vi "AfterLoad.vi"(8 "error in (no error)":errorcluster, 11 "SettingsFile in":refnum<class "SettingsFile.lvclass">) -> (0 "error out":errorcluster, 3 "SettingsFile out":refnum<class "SettingsFile.lvclass">)   [LabVIEW 2018, in "SettingsFile.lvclass"]
uses:
  SettingsFile.lvclass
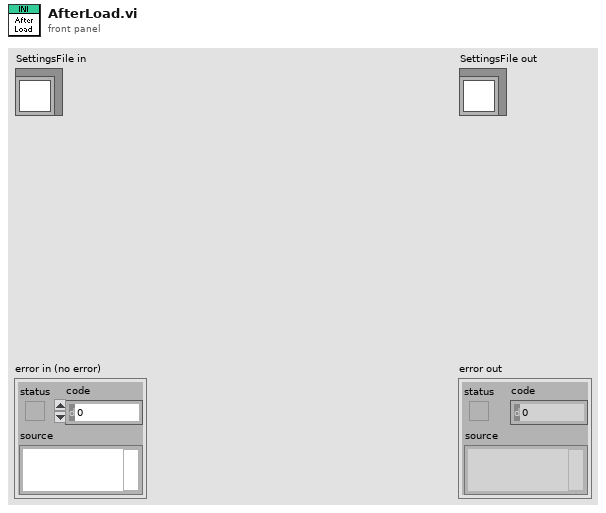
[diagram p1: front panel]
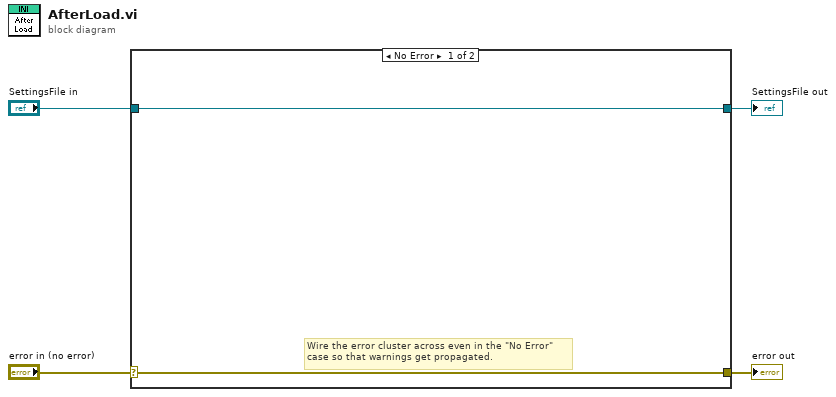
[diagram p0: block diagram]
diagram:
  n1 = case shown="No Error" "error in (no error)" {
    selector: "error in (no error)" -> [w5 w8]
    tunnel: [w5 w8] -> w3
    tunnel: [w6 w7] -> w1
    tunnel: "SettingsFile in" -> [w6 w7]
    frame No Error {
      # "Wire the error cluster across even in the \"No Error\"\ncase so that warnings get propagated."
    }
    frame Error {
    }
  }
  "error out" <- w3
  "SettingsFile out" <- w1
